vi "RichToFlatnixnet_grpc_GetSubPropertyRequest.vi"(5 "OutputClusterType":T1, 11 "InputCluster":T4) -> (3 "OutputCluster":T1)   [LabVIEW 2025, in "grpc-xnet_client.lvlib"]
uses:
  grpc-xnet_client.lvlib
  nixnet_grpc_GetSubPropertyRequest.ctl
  nixnet_grpc_GetSubPropertyRequest_subproperty_id_enum/nixnet_grpc_GetSubPropertyRequest_subproperty_id_enum.lvclass
  nidevice_grpc_Session.ctl
  nixnet_grpc_GetSubPropertyRequest_Flat.ctl
  nidevice_grpc_Session_Flat.ctl
  nixnet_grpc_SubProperty.ctl
  nixnet_grpc_GetSubPropertyRequest_subproperty_id_enum/nixnet_grpc_GetSubPropertyRequest_subproperty_id_enum.lvclass/nixnet_grpc_GetSubPropertyRequest_subproperty_id_enum.ctl
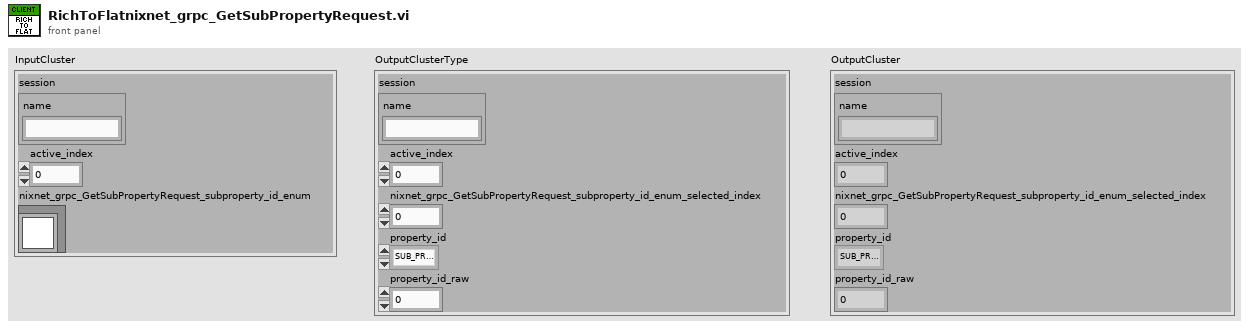
[diagram p1: front panel]
types:
  T1 = typedef "grpc-xnet_client.lvlib/nixnet_grpc_GetSubPropertyRequest_Flat.ctl" = cluster{"session":T2, "active_index":u32, "nixnet_grpc_GetSubPropertyRequest_subproperty_id_enum_selected_index":i32, "property_id":T3, "property_id_raw":u32}
  T2 = typedef "grpc-xnet_client.lvlib/nidevice_grpc_Session_Flat.ctl" = cluster{"name":string}
  T3 = typedef "grpc-xnet_client.lvlib/nixnet_grpc_SubProperty.ctl" = enum32{"SUB_PROPERTY_UNSPECIFIED", "SUB_PROPERTY_SESSION_SUB_CAN_START_TIME_OFF", "SUB_PROPERTY_SESSION_SUB_CAN_TX_TIME", "SUB_PROPERTY_SESSION_SUB_LIN_TX_N_CORRUPTED_CHKSUMS", "SUB_PROPERTY_SESSION_SUB_OUTPUT_QUEUE_UPDATE_FREQ", "SUB_PROPERTY_SESSION_SUB_J1939_ADDR_FILTER", "SUB_PROPERTY_SESSION_SUB_SKIP_N_CYCLIC_FRAMES"}
  T4 = typedef "grpc-xnet_client.lvlib/nixnet_grpc_GetSubPropertyRequest.ctl" = cluster{"session":T5, "active_index":u32, "nixnet_grpc_GetSubPropertyRequest_subproperty_id_enum":refnum<class "nixnet_grpc_GetSubPropertyRequest_subproperty_id_enum.lvclass">}
  T5 = typedef "grpc-xnet_client.lvlib/nidevice_grpc_Session.ctl" = cluster{"name":string}
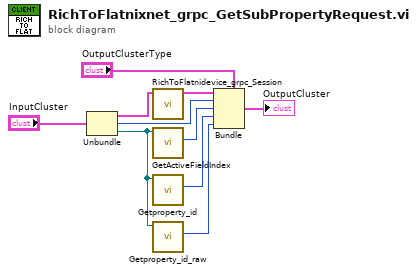
[diagram p0: block diagram]
diagram:
  n1 = Unbundle "Unbundle"("InputCluster") -> ("session"=w7:T5, "active_index"=w5:u32, "nixnet_grpc_GetSubPropertyRequest_subproperty_id_enum"=w4:refnum<class "nixnet_grpc_GetSubPropertyRequest_subproperty_id_enum.lvclass">)
  n2 = call "RichToFlatnidevice_grpc_Session.vi"("InputCluster"=w7) -> ("OutputCluster"=w6:T2)  [unwired: 10 in]
  n3 = call "GetActiveFieldIndex.vi"("OneOfTemplate in"=w4) -> ("Active Field Index"=w3:i32)  [unwired: 8 in, 2 out]
  n4 = call "Getproperty_id.vi"("OneOfTemplate in"=w4) -> ("Get_Val"=w2:T3)  [unwired: 8 in, 2 out]
  n5 = call "Getproperty_id_raw.vi"("OneOfTemplate in"=w4) -> ("Get_Val"=w1:u32)  [unwired: 8 in, 2 out]
  n6 = Bundle "Bundle"(cluster="OutputClusterType", "session"=w6, "active_index"=w5, "nixnet_grpc_GetSubPropertyRequest_subproperty_id_enum_selected_index"=w3, "property_id"=w2, "property_id_raw"=w1) -> (→"OutputCluster":T1)
